vi "slapmiDataStream.vi"() -> ()   [LabVIEW 2015]
doc: "Use this VI as a template for the reconfigurable oscilloscope streaming acquisition design. The block diagram is divided into two main loops: the Register Bus loop and the Acquisition loop.\n\n<B>Register Bus</B>: This loop initializes the registers that are needed to support the configuration of the device. The FIFO bus, on the left, allows all the other design libraries to communicate with one another. This loop is very important to support the proper behavior of the design library components.\n\n<B>Acquisition</B>: Acquires data from the I/O channels and writes the data into the DMA FIFO. Before writing to the DMA FIFO, the data is written to and read from a DRAM FIFO. The purpose of the DRAM FIFO is to provide a data buffer to guard against buffer overrun of the DMA FIFO. The DMA FIFO transmits the data to the Fetch VIs on the host. This VI also evaluates the various acquisition triggers."
uses:
  Typedefs/StateMachineStates.ctl
  <vilib>/Platform/TimedLoop/XDataNode/timing_clust.ctl
  <vilib>/Platform/TimedLoop/XDataNode/nitl_modes.ctl
  <vilib>/Platform/TimedLoop/XDataNode/wakeup.ctl
  <vilib>/rvi/Emulation/niFpgaSctlEmulationGetInTimedLoop.vi
  <vilib>/rvi/Emulation/niFpgaEmulationReportErrorSimple.vi
  <vilib>/rvi/Emulation/niFpgaGetClockAttributes.vi
  <vilib>/rvi/Emulation/niFpgaCriticalErrorInLSC.vi
  <vilib>/rvi/eio/common/nirviEmuTemplateMethod_errors.vi
  SubVIs/Data Type Conversion/SubVIs/Data Type Conversion FXP(+-,18,1) to I16x8ch.vi
  <instrlib>/HSAI-RIO/Config/Group A/v1/FPGA/Digital Correction/Validate 8 Channel Data.vi
  <instrlib>/HSAI-RIO/Config/Group A/v1/FPGA/Digital Correction/Digital Correction (8 Ch).vi
  <vilib>/Platform/TimedLoop/XDataNode/XDataNode.xnode
  <vilib>/eio/EIONode/EIONode.xnode
  <vilib>/Platform/TimedLoop/XDataNode/XDNodeRunTimeDep.lvlib
  <instrlib>/_niInstr/FIFO Register Bus/v1/FPGA/niInstr FIFO Register Bus v1 FPGA.lvclass
  <instrlib>/_niInstr/Instruction Framework/v1/FPGA/Top Level Bus/Register Configuration/Register Configuration.lvclass
  <instrlib>/HSAI-RIO/Config/Group A/v1/FPGA/Digital Correction/Digital Correction.lvclass
  <instrlib>/HSAI-RIO/Config/Group A/v1/FPGA/Config Registers/Config Registers.lvclass
panel:
  in  "Ref Clk Decimation":u8=25
  out "AliveCtr":u16
  in  "Num Slices":u16
  in  "Frame Clock Period":u64
  in  "LaserClkDelay":u8
  out "Galvo6RawPos":i16
  out "Galvo5RawPos":i16
  out "GalvoSamplesRemaining":u32
  in  "GalvoRecordDecimation":u32
  in  "GalvoRecordSamples":u32
  in  "GalvoRecordArm":bool
  in  "Reset":bool
  out "AcqStatus":T1
  in  "EnableGalvoDataStream":bool
  in  "EnableRawDataStream":bool
  out "FrameTagFifoTimeouts":u64
  out "ShortPmtDataFifoTimeouts":u64
  in  "SamplesPerLaserClk":u8
  in  "Enable":bool
  out "FramesDone":u32
  in  "Abort":bool
  in  "FramesToCollect":u32
  in  "PXITrigExtStartTrig":u8
  in  "PXITrigLaserClk":u8
  out "GalvoDataFifoTimeouts":u64
  out "PmtDataFifoTimeouts":u64
  in  "AcqSoftStartTrig":bool
  out "Pmt1RawData":i16
  out "Pmt2RawData":i16
  out "Galvo4RawPos":i16
  out "Galvo3RawPos":i16
  out "Galvo2RawPos":i16
  out "Galvo1RawPos":i16
  out "fifo reg bus data 0":u64
  out "fifo reg bus status 0":u32
  in  "fifo reg bus ctrl 0":u32
  # "Configuration Register Bus Controls"
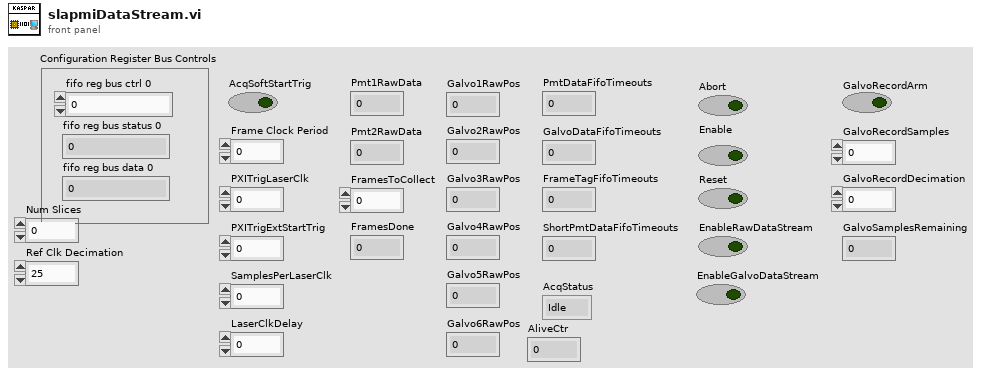
[diagram p1: front panel]
types:
  T1 = typedef "StateMachineStates.ctl" = enum16{"Idle", "Armed", "Running", "Galvo Record Armed", "Galvo Recording"}
  T2 = typedef "XDNodeRunTimeDep.lvlib/timing_clust.ctl" = cluster{"Expected End [f-1]":u64, "Actual End [f-1]":u64, "Finished Late? [f-1]":bool, "Expected End [i-1]":u64, "Actual End [i-1]":u64, "Finished Late? [i-1]":bool, "Expected Start [i]":u64, "Actual Start [i]":u64, "Expected Start [f]":u64, "Actual Start [f]":u64, "Source Name":string, "Structure Name":string, "Period":i64, "Deadline":i64, "Offset":i64, "Start":i64, "Priority":i32, "Timeout":i32, "Mode":T3, "Wakeup Reason":T4, "Error":errorcluster, "Source Type":string, "Secondary Source Type":string, "Global End Time":u64, "Global Start Time":u64, "Frame Duration":u64, "Iteration Duration":u64, "Assigned CPU":i32, "I/O Scan Engine Mode":u32}
  T3 = typedef "XDNodeRunTimeDep.lvlib/nitl_modes.ctl" = enum32{"No Change", "Process missed periods, maintain original phase", "Discard missed periods, maintain original phase", "Process missed periods, ignore original phase", "Discard missed periods, ignore original phase"}
  T4 = typedef "XDNodeRunTimeDep.lvlib/wakeup.ctl" = enum32{"Normal", "Aborted", "Asynchronous wakeup", "Timing source error", "Timed loop error", "Timeout"}
  T5 = cluster{"Channel 0":fxp<+/-,14,1>[], "Channel 1":fxp<+/-,14,1>[], "Channel 2":fxp<+/-,14,1>[], "Channel 3":fxp<+/-,14,1>[], "Channel 4":fxp<+/-,14,1>[], "Channel 5":fxp<+/-,14,1>[], "Channel 6":fxp<+/-,14,1>[], "Channel 7":fxp<+/-,14,1>[]}
  T6 = cluster{"Channel 0":fxp<+/-,18,1>[], "Channel 1":fxp<+/-,18,1>[], "Channel 2":fxp<+/-,18,1>[], "Channel 3":fxp<+/-,18,1>[], "Channel 4":fxp<+/-,18,1>[], "Channel 5":fxp<+/-,18,1>[], "Channel 6":fxp<+/-,18,1>[], "Channel 7":fxp<+/-,18,1>[]}
  T7 = cluster{"GalvoRecordArm":bool, "GalvoRecordSamples":u32, "GalvoRecordDecimation":u32}
  T8 = cluster{"channel 0":i16[], "channel 1":i16[], "channel 2":i16[], "channel 3":i16[], "channel 4":i16[], "channel 5":i16[], "channel 6":i16[], "channel 7":i16[]}
  T9 = cluster{"SamplesPerLaserClk":u8, "Frame Clock Period":u64, "Num Slices":u16, "Enable":bool, "Reset":bool, "Abort":bool}
  T10 = typedef "AcqStatus.ctl" = cluster{"AcqStatusRunning":bool, "AcqStatusClock":u64, "LaserPulse":bool, "AcqReset":bool, "LaserClcksLastFrame":u32, "SamplesLastFrame":u32, "WriteFrameTag":bool, "WriteShortPulseSample":bool, "Frames Done":u32, "GalvoRecordMode":bool}
  T11 = cluster{"Galvo1RawPos":i16, "Galvo2RawPos":i16, "Galvo3RawPos":i16, "Galvo4RawPos":i16, "Galvo5RawPos":i16, "Galvo6RawPos":i16}
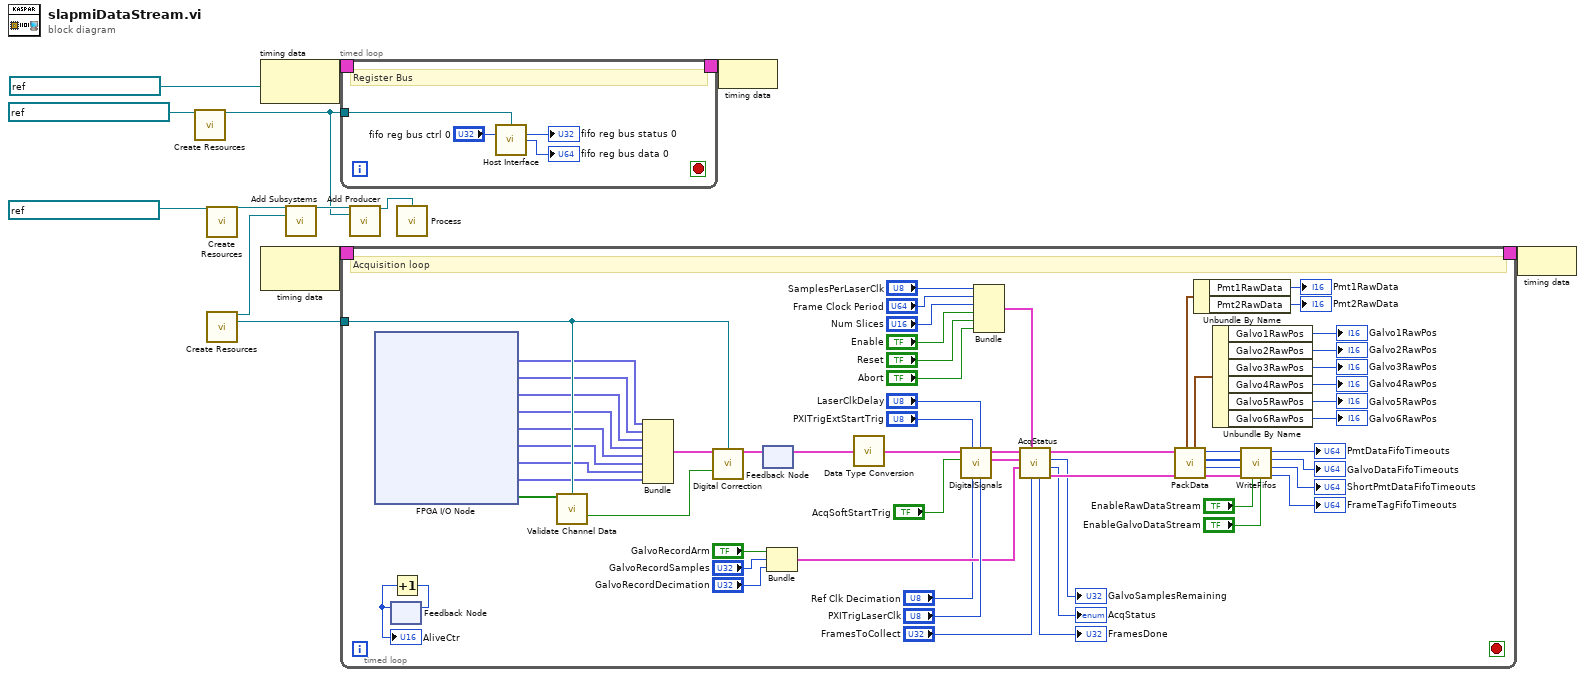
[diagram p0: block diagram]
diagram:
  n1 = call <instrlib>:"Create Resources.vi"("instruction fifo"=refnum<k21> "reg.host instruction fifo 0" ("FIFO")) -> ("fifo register bus"=w2:refnum<class "niInstr FIFO Register Bus v1 FPGA.lvclass">)  [unwired: 14 in]
  n2 = call <instrlib>:"Create Resources.vi"("register clock"=refnum<k21> "40 MHz Onboard Clock" ("Source Name")) -> ("register configuration"=w5:refnum<class "Register Configuration.lvclass">)  [unwired: 14 in]
  n3 = call <instrlib>:"Create Resources.vi"() -> ("config subsystems"=w4:refnum<class "Address Space Collection.lvclass">, "digital correction resources"=w7:refnum<class "Digital Correction.lvclass">)  [unwired: 14 in]
  n4 = node-c288(refnum<k21> "40 MHz Onboard Clock" ("Source Name")) -> (w13:T2)
  n5 = node-c288() -> (w11:T2)  [unwired: 1 in]
  n6 = call <instrlib>:"Add Subsystems.vi"("register configuration in"=w5, "subsystems"=w4) -> ("register configuration out"=w3:refnum<class "Register Configuration.lvclass">)  [unwired: 13 in]
  n7 = timed-loop {
    timing: w13 -> [_]
    timing-out: [_] -> w12
    tunnel: w2 -> [w17]
    stop <- _ stop-if-true
    # "Register Bus"
    n8 = call <instrlib>:"Host Interface.vi"("fifo register bus"=w17, "fifo reg bus ctrl 0"="fifo reg bus ctrl 0") -> ("fifo reg bus status 0"=→"fifo reg bus status 0":u32, "fifo reg bus data 0"=→"fifo reg bus data 0":u64)  [unwired: 12 in]
  }
  n9 = timed-loop {
    timing: w11 -> [_]
    timing-out: [_] -> w10
    tunnel: w7 -> [w80]
    stop <- _ stop-if-true
    # "Acquisition loop"
    n10 = xnode "FPGA I/O Node"() -> ("Channel 0"=w76:fxp<+/-,14,1>[], "Channel 1"=w77:fxp<+/-,14,1>[], "Channel 2"=w78:fxp<+/-,14,1>[], "Channel 3"=w79:fxp<+/-,14,1>[], "Channel 4"=w73:fxp<+/-,14,1>[], "Channel 5"=w72:fxp<+/-,14,1>[], "Channel 6"=w71:fxp<+/-,14,1>[], "Channel 7"=w70:fxp<+/-,14,1>[], "Channel Data Valid"=w67:bool[])  [unwired: 9 in, 9 out]
    n11 = feedback #1() -> (w21:u16)  [unwired: 1 in]
    "AliveCtr" <- w21
    n12 = Increment(x=w21) -> (x+1=w22:u16)
    n13 = feedback-in #1(w22) -> ()
    n14 = call-poly <instrlib>:"Validate Channel Data.vi"("channel data valid"=w67, "digital correction resources"=w80) -> ("expected data valid"=w75:bool)  [unwired: 13 in]
    n15 = Bundle("Channel 0"=w76, "Channel 1"=w77, "Channel 2"=w78, "Channel 3"=w79, "Channel 4"=w73, "Channel 5"=w72, "Channel 6"=w71, "Channel 7"=w70) -> (w69:T5)  [unwired: 1 in]
    n16 = call-poly <instrlib>:"Digital Correction.vi"("channel data in"=w69, "digital correction resources"=w80, "input valid"=w75) -> ("corrected channel data out"=w74:T6)  [unwired: 11 in, 1 out]
    n17 = feedback #2() -> (w68:T6)  [unwired: 1 in]
    n18 = feedback-in #2(w74) -> ()
    n19 = Bundle("GalvoRecordArm"="GalvoRecordArm", "GalvoRecordSamples"="GalvoRecordSamples", "GalvoRecordDecimation"="GalvoRecordDecimation") -> (w35:T7)  [unwired: 1 in]
    n20 = call-poly "Data Type Conversion.vi"("data in"=w68) -> ("data out"=w48:T8)  [unwired: 3 in, 1 out]
    n21 = call "DigitalSignals.vi"("PXITrigLaserClk"="PXITrigLaserClk", "LaserClkDelay"="LaserClkDelay", "Ref Clk Decimation"="Ref Clk Decimation", "PXITrigExtStartTrig"="PXITrigExtStartTrig", "AcqSoftStartTrig"="AcqSoftStartTrig", "data in"=w48) -> ("Digital Signals"=w25:cluster{"StartTrig":bool, "LaserClk":bool}, "data out"=w47:T8)  [unwired: 4 in]
    n22 = Bundle("SamplesPerLaserClk"="SamplesPerLaserClk", "Frame Clock Period"="Frame Clock Period", "Num Slices"="Num Slices", "Enable"="Enable", "Reset"="Reset", "Abort"="Abort") -> (w24:T9)  [unwired: 1 in]
    n23 = call "AcqStatus.vi"("FramesToCollect"="FramesToCollect", "Acq Params"=w24, "Galvo Record"=w35, "Digital Signals"=w25, "data in"=w47) -> ("AcqStatus"=w56:T10, "AcqSatus"=→"AcqStatus":T1, "GalvoSamplesRemaining"=→"GalvoSamplesRemaining":u32, "data out"=w57:T8, "FramesDone"=→"FramesDone":u32)  [unwired: 2 in]
    n24 = call "PackData.vi"("AcqStatusIn"=w56, "data in"=w57) -> ("AcqStatusOut"=w54:T10, "FrameTagDataPack"=w45:u64, "GalvoDataPack"=w58:u64[], "PmtDataPack"=w55:u64, "GalvoData"=w59:T11, "PmtData"=w62:cluster{"Pmt1RawData":i16, "Pmt2RawData":i16})  [unwired: 4 in]
    n25 = Unbundle By Name(w62) -> ("Pmt1RawData"=→"Pmt1RawData":i16, "Pmt2RawData"=→"Pmt2RawData":i16)
    n26 = Unbundle By Name(w59) -> ("Galvo1RawPos"=→"Galvo1RawPos":i16, "Galvo2RawPos"=→"Galvo2RawPos":i16, "Galvo3RawPos"=→"Galvo3RawPos":i16, "Galvo4RawPos"=→"Galvo4RawPos":i16, "Galvo5RawPos"=→"Galvo5RawPos":i16, "Galvo6RawPos"=→"Galvo6RawPos":i16)
    n27 = call "WriteFifos.vi"("EnableGalvoDataStream"="EnableGalvoDataStream", "EnableRawDataStream"="EnableRawDataStream", "AcqStatusOut"=w54, "FrameTagDataPack"=w45, "GalvoDataPack"=w58, "PmtDataPack"=w55) -> ("FrameTagFifoTimeouts"=→"FrameTagFifoTimeouts":u64, "ShortPmtDataFifoTimeouts"=→"ShortPmtDataFifoTimeouts":u64, "GalvoDataFifoTimeouts"=→"GalvoDataFifoTimeouts":u64, "PmtDataFifoTimeouts"=→"PmtDataFifoTimeouts":u64)  [unwired: 2 in]
  }
  n28 = call <instrlib>:"Add Producer.vi"("register configuration in"=w3, "instruction producer"=w2) -> ("register configuration out"=w1:refnum<class "Register Configuration.lvclass">)  [unwired: 13 in]
  n29 = call <instrlib>:"Process.vi"("register configuration"=w1) -> ()  [unwired: 15 in]
  n30 = node-c288(w12) -> ()
  n31 = node-c288(w10) -> ()
